vi "Item_Init.vi"(11 "Object":T1) -> ()   [LabVIEW 2019, in "BlueSerializationProvider.lvlib"]
uses:
  BlueSerializationProvider.lvlib
  <resource>/Framework/Providers/API/ItemRef.ctl
panel:
  out "error out":errorcluster
  in  "error in":errorcluster
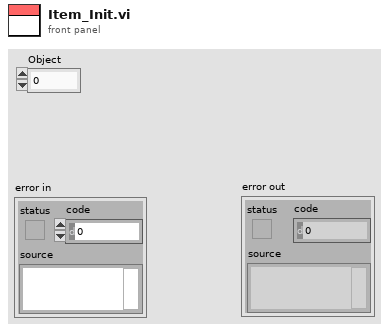
[diagram p1: front panel]
types:
  T1 = typedef "ItemRef.ctl" = u64
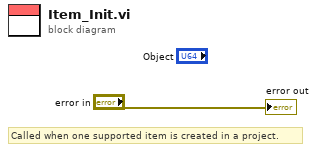
[diagram p0: block diagram]
diagram:
  # "Called when one supported item is created in a project."
  "error out" <- "error in"
